vi "Add Test Event.vi"(8 "error in (no error)":errorcluster, 10 "Test Assert Event":T1={"Name"="", "Passed"=FALSE, "Call Chain"=[], "Test Error"={"status"=FALSE, "code"=0, "source"=""}, "Time Stamp"=timestamp(0 s since 1904-01-01), "Unique Assert ID"="", "Test ID"="", "Execution time (s)"=-1.0, "Verbose Explanation"=""}, 11 "Test Event Storage in":refnum<class "Test Event Storage.lvclass">) -> (0 "error out":errorcluster, 2 "Assert ID":string, 3 "Test Event Storage out":refnum<class "Test Event Storage.lvclass">)   [LabVIEW 2013, in "Caraya.lvlib" / "Test Event Storage.lvclass"]
uses:
  Test Event Storage.lvclass
  Test Result/Assert Event Data.ctl
  Test Event Storage.lvclass/Test Event Storage.ctl
  Test Result/Test Result.lvclass
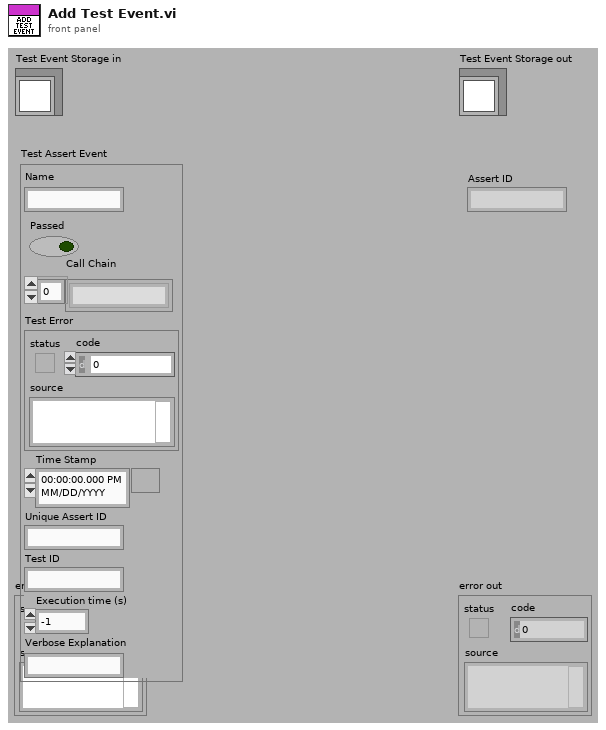
[diagram p1: front panel]
types:
  T1 = typedef "Caraya.lvlib/Test Result.lvclass/Assert Event Data.ctl" = cluster{"Name":string, "Passed":bool, "Call Chain":string[], "Test Error":errorcluster, "Time Stamp":timestamp, "Unique Assert ID":string, "Test ID":string, "Execution time (s)":dbl, "Verbose Explanation":string}
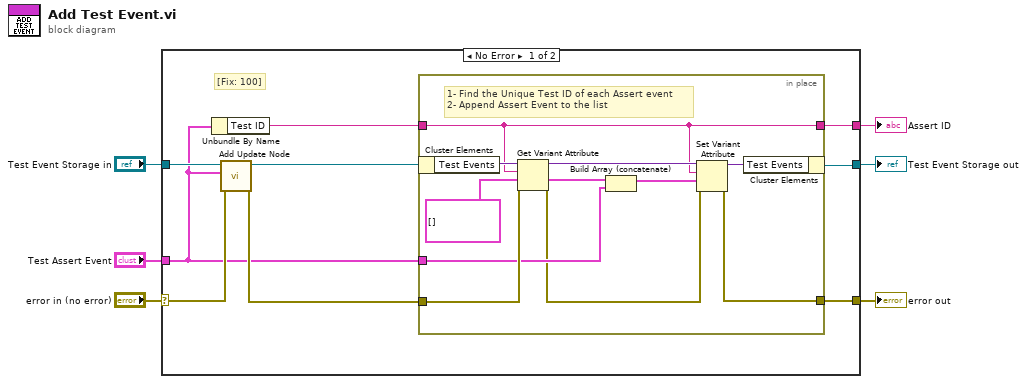
[diagram p0: block diagram]
diagram:
  n1 = case shown="No Error" "error in (no error)" {
    selector: "error in (no error)" -> [w10 w28]
    tunnel: [w15 w28] -> w5
    tunnel: [w14 w27] -> w3
    tunnel: "Test Event Storage in" -> [w13 w27]
    tunnel: "Test Assert Event" -> [w7 _]
    tunnel: [w8 _] -> w1
    frame No Error {
      # "[Fix: 100]"
      n2 = Unbundle By Name(w7) -> ("Test ID"=w9:string)
      n3 = call "Add Update Node.vi"("error in (no error)"=w10, "Test Event"=w7, "Test Event Storage in"=w13) -> ("error out"=w11:errorcluster, "Test Event Storage out"=w12:refnum<class "Test Event Storage.lvclass">)  [unwired: 6 in, 1 out]
      n4 = in-place {
        in-place-border: w11 -> [w23]
        in-place-border: w9 -> [w17]
        in-place-border: w7 -> [w21]
        in-place-border: [w19] -> w15
        in-place-border: [w17] -> w8
        # "1- Find the Unique Test ID of each Assert event\n2- Append Assert Event to the list"
        n5 = in-place-cluster #1(w12) -> ("Test Events"=w26:variant)
        n6 = Get Variant Attribute(Variant=w26, name=w17, default value (empty Variant)=T1[] [], error in=w23) -> (duplicate Variant=w24:variant, value=w22:T1[], error out=w18:errorcluster)  [unwired: 1 out]
        n7 = Build Array (concatenate)(w22, w21) -> (w20:T1[])
        n8 = Set Variant Attribute(Variant=w24, name=w17, value=w20, error in=w18) -> (Variant out=w25:variant, error out=w19:errorcluster)  [unwired: 1 out]
        n9 = in-place-cluster #1("Test Events"=w25) -> (w14:refnum<class "Test Event Storage.lvclass">)
      }
    }
    frame Error {
    }
  }
  "error out" <- w5
  "Test Event Storage out" <- w3
  "Assert ID" <- w1
